vi "Scott -- strain -- voltage-wave-form-generator.vi"(6 "index":i32, 7 "voltage-wave-control":T1=enum."next", 11 "voltage-parameters-IN":T2) -> (0 "voltage out (V)":dbl, 2 "time (sec) out":dbl, 3 "voltage-parameters OUT":T2)   [LabVIEW 2014]
uses:
  Scott -- strain -- voltage-wave-generator-parameters.ctl
  FSU/ScottRiggs/Piezo/votage-control.ctl
  FSU/ScottRiggs/Piezo2/voltage-wave-generator-parameters.ctl
  Q - not nan -- real.vi
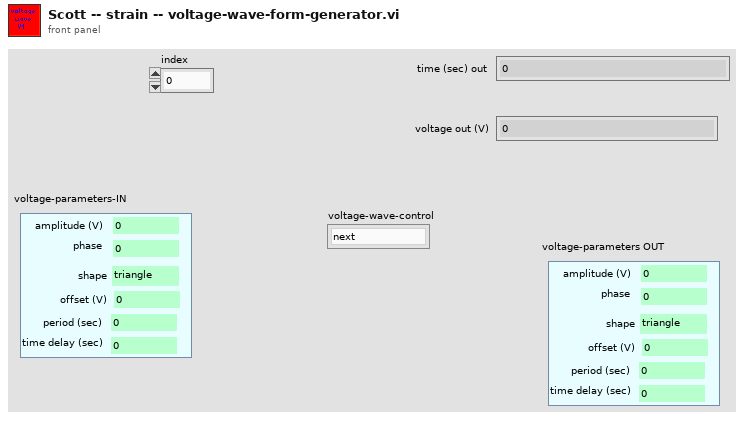
[diagram p1: front panel]
types:
  T1 = typedef "votage-control.ctl" = enum16{"reset", "next", "use index"}
  T2 = typedef "Scott -- strain -- voltage-wave-generator-parameters.ctl" = cluster{"phase ":dbl, "amplitude (V)":dbl, "offset (V)":dbl, "time delay (sec)":dbl, "period (sec)":dbl, "shape":enum16{"triangle", "sine", "none"}}
  T3 = typedef "voltage-wave-generator-parameters.ctl" = cluster{"phase ":dbl, "amplitude (V)":dbl, "offset (V)":dbl, "time delay (sec)":dbl, "period (sec)":dbl, "shape":enum16{"triangle", "sine", "none"}}
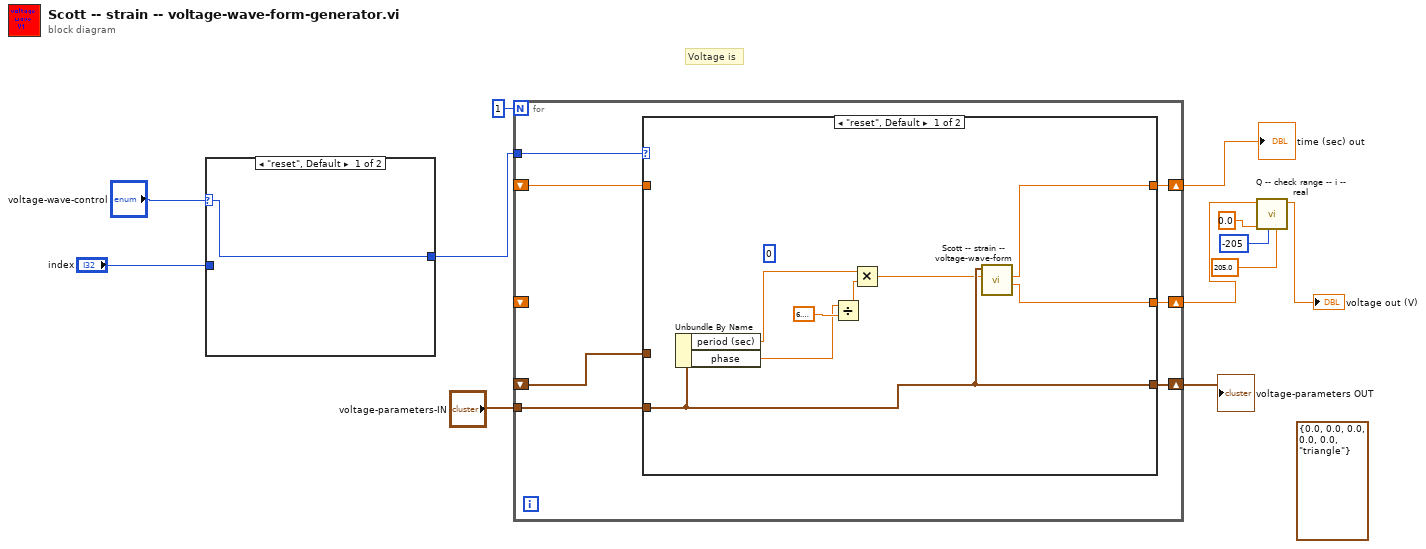
[diagram p0: block diagram]
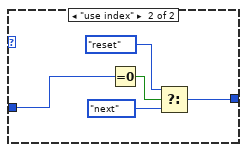
[diagram p2: hidden frame]
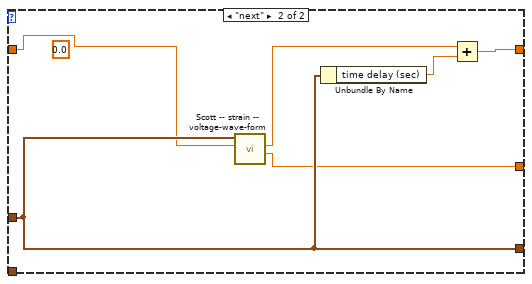
[diagram p3: hidden frame]
diagram:
  (unwired) T3 {"phase "=0.0, "amplitude (V)"=0.0, "offset (V)"=0.0, "time delay (sec)"=0.0, "period (sec)"=0.0, "shape"=enum."triangle"} ("Cluster")
  # "Voltage is"
  n1 = case shown="\"reset\", Default" "voltage-wave-control" {
    selector: "voltage-wave-control" -> [w13 _]
    tunnel: "index" -> [_ w15]
    tunnel: [w13 w14] -> w1
    frame "reset", Default {
    }
    frame "use index" {
      n2 = Equal To 0?(x=w15) -> (x = 0?=w18:bool)
      n3 = Select(t=votage-control."reset" ("voltage-wave-control"), s=w18, f=votage-control."next" ("voltage-wave-control")) -> (s? t:f=w14:T1)
    }
  }
  n4 = for {
    N: 1 -> [_]
    tunnel: w1 -> [w25]
    tunnel: "voltage-parameters-IN" -> [w24]
    shift-right: [w23] -> w10
    shift-left: _ -> [w22]
    shift-right: [w21] -> w11
    shift-left: _ -> [w20]
    shift-right: [w19] -> w6
    shift-left: _ -> [_]
    n5 = case shown="\"reset\", Default" w25 {
      tunnel: w24 -> [w28 _]
      tunnel: [w28 w37] -> w23
      tunnel: w22 -> [_ w37]
      tunnel: [w26 w39] -> w21
      tunnel: w20 -> [_ w36]
      tunnel: [w29 w35] -> w19
      frame "reset", Default {
        (unwired) 0
        n6 = Unbundle By Name(w28) -> ("period (sec)"=w30:dbl, "phase"=w32:dbl)
        n7 = Divide(x=w32, y=6.283185307179586) -> (x/y=w31:dbl)
        n8 = Multiply(x=w30, y=w31) -> (x*y=w27:dbl)
        n9 = call "Scott -- strain -- voltage-wave-form.vi"("time (sec)"=w27, "voltage-parameters-IN"=w28) -> ("voltage"=w29:dbl, "time (sec) out"=w26:dbl)  [unwired: 8 in]
      }
      frame "next" {
        (unwired) 0.0
        n10 = call "Scott -- strain -- voltage-wave-form.vi"("time (sec)"=w36, "voltage-parameters-IN"=w37) -> ("voltage"=w35:dbl, "time (sec) out"=w34:dbl)  [unwired: 8 in]
        n11 = Unbundle By Name(w37) -> ("time delay (sec)"=w38:dbl)
        n12 = Add(x=w34, y=w38) -> (x+y=w39:dbl)
      }
    }
  }
  "time (sec) out" <- w11
  "voltage-parameters OUT" <- w10
  n13 = call "Q -- check range -- i -- real.vi"("upper"=205.0, "lower"=-205, "default"=0.0, "number"=w6) -> ("number in range"=→"voltage out (V)":dbl)  [unwired: 5 in, 2 out]
